vi "Message Handling Loop - UI.vi"(8 "error in":errorcluster, 9 "UI":refnum<queue>, 10 "User Event Bundle":T1) -> (0 "error out":errorcluster)   [LabVIEW 2018]
uses:
  Type Defs/Filter Cluster.ctl
  Support/Message Queue/Message Queue.lvlib
  Support/Message Queue/Enqueue Message (Single).vi
  <vilib>/Utility/error.llb/Error Cluster From Error Code.vi
  <vilib>/ErrorRing/Error Ring.xnode
  Type Defs/UI Loop Data.ctl
  Type Defs/Sorting Methods.ctl
  Type Defs/SR Cluster.ctl
  Type Defs/SR Status.ctl
  Support/User Events/User Events.lvlib
  Support/Message Queue/Message Cluster.ctl
  Type Defs/User Events.ctl
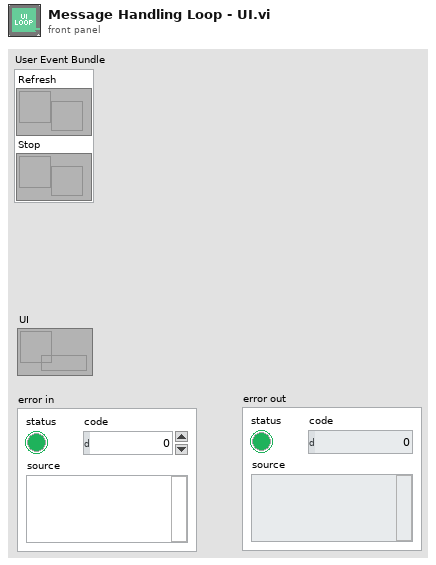
[diagram p1: front panel]
types:
  T1 = typedef "User Events.ctl" = cluster{"Refresh":refnum<user-event>, "Stop":refnum<user-event>}
  T2 = typedef "UI Loop Data.ctl" = cluster{"SR Display List":T3[], "Filter Cluster":T5, "Exit":refnum<vi>, "Main VI":refnum<vi>, "Sorting":T6, "SR Display List":refnum<vi>}
  T3 = typedef "SR Cluster.ctl" = cluster{"Color":u32, "SR Number":i32, "SR Status":T4, "Name":string, "Summary":string, "Last Updated":timestamp, "SR Type":string, "Service Level":string, "Days Open":dbl, "Creation Date":timestamp}
  T4 = typedef "SR Status.ctl" = enum16{"Caller Abandoned", "Created in Error", "Expired", "Forum Resolved AE", "Forum Resolved Customer", "IN WORK", "IN WORK Collab with AES", "IN WORK Collab with PSE", "IN WORK Collab with SE", "IN WORK Customer Added Note", "IN WORK Escalation", "IN WORK Wait on Customer", "Open", "Potentially Resolved", "Presumed Resolved", "RMA Approved for Return", "Resolved", "Passed Off"}
  T5 = typedef "Filter Cluster.ctl" = cluster{"Show Resolved":bool, "Show Potentially Resolved":bool, "Show Passoffs":bool, "Show In Collab":bool}
  T6 = typedef "Sorting Methods.ctl" = enum16{"SR Status", "Most Recent", "SR Type", "SR Number"}
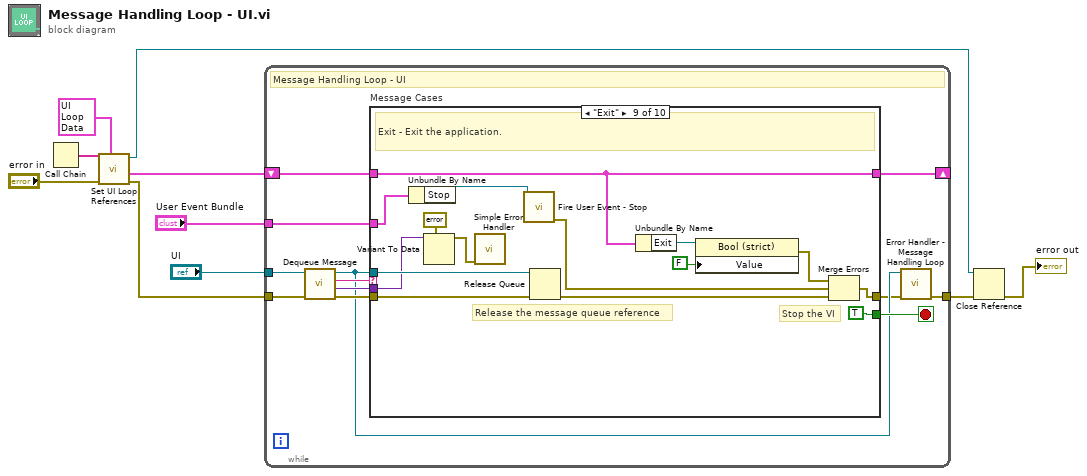
[diagram p0: block diagram]
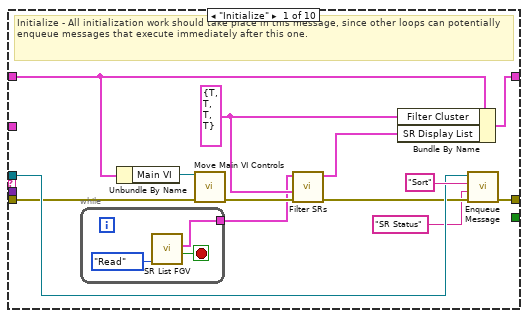
[diagram p2: hidden frame]
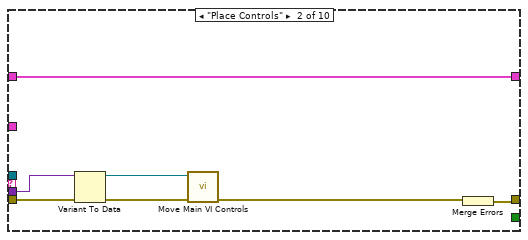
[diagram p3: hidden frame]
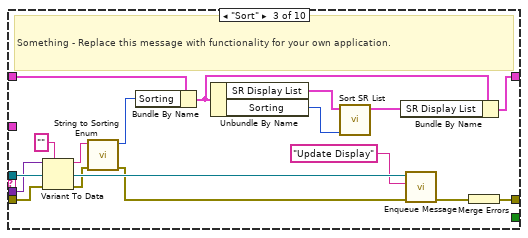
[diagram p4: hidden frame]
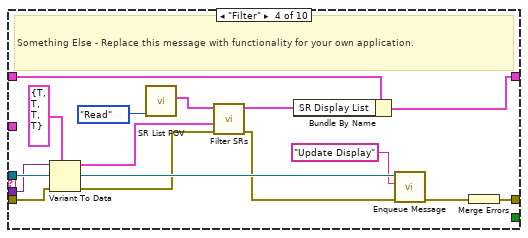
[diagram p5: hidden frame]
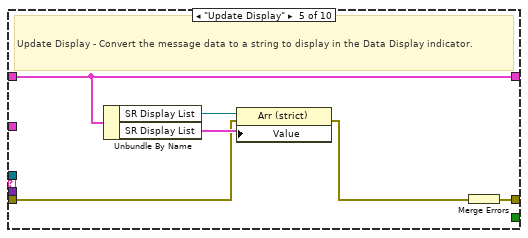
[diagram p6: hidden frame]
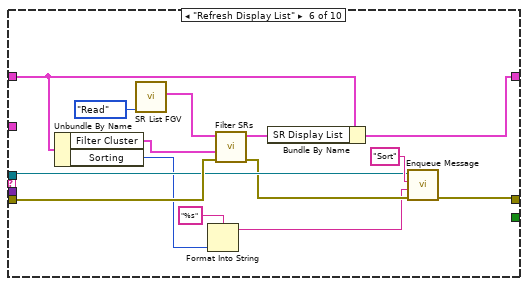
[diagram p7: hidden frame]
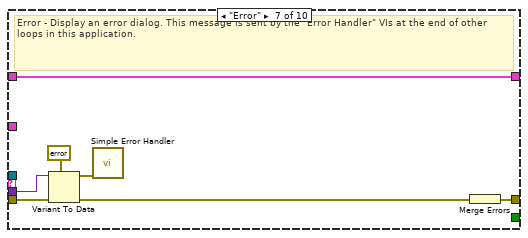
[diagram p8: hidden frame]
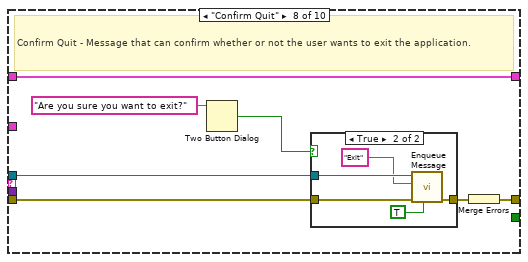
[diagram p9: hidden frame]
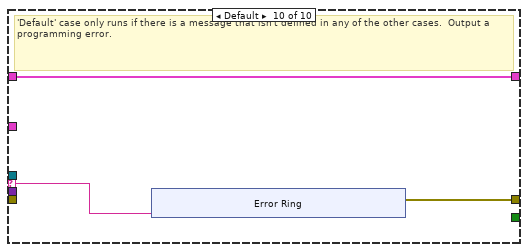
[diagram p11: hidden frame]
diagram:
  n1 = Call Chain() -> (call chain=w4:string[])
  n2 = call "Set UI Loop References.vi"("UI Data in"=T2 {"SR Display List"=[], "Filter Cluster"={"Show Resolved"=TRUE, "Show Potentially Resolved"=TRUE, "Show Passoffs"=TRUE, "Show In Collab"=TRUE}, "Exit"=refnum, "Main VI"=refnum, "Sorting"=enum."SR Status", "SR Display List"=refnum}, "error in (no error)"="error in", "call chain"=w4) -> ("error out"=w8:errorcluster, "UI Data out"=w9:T2, "VI reference out"=w7:refnum<vi>)  [unwired: 6 in]
  n3 = while {
    tunnel: "UI" -> [w15]
    shift-right: [w21] -> _
    shift-left: w9 -> [w22]
    tunnel: w8 -> [w19]
    tunnel: [w13] -> w5
    tunnel: "User Event Bundle" -> [w11]
    stop <- w20 stop-if-true
    # "Message Handling Loop - UI"
    n4 = call "Dequeue Message.vi"("error in (no error)"=w19, "Message Queue"=w15) -> ("error out"=w18:errorcluster, "Message Data"=w16:variant, "Message"=w17:string, "dup Message Queue"=w14:refnum<queue>)  [unwired: 6 in]
    n5 = case "Message Cases" shown="\"Exit\"" w17 {
      selector: w17 -> [_ _ _ _ _ _ _ _ _ w133]
      tunnel: w14 -> [w33 _ w60 w75 _ w91 _ w107 w132 _]
      tunnel: w18 -> [w32 w44 w55 w65 w79 w93 w104 w111 w129 _]
      tunnel: [w35 w40 w62 w77 w83 w89 w98 w109 w122 w134] -> w12
      tunnel: w22 -> [w30 w45 w48 w70 w82 w88 w103 w110 w125 w135]
      tunnel: [w31 w45 w57 w68 w82 w94 w103 w110 w125 w135] -> w21
      tunnel: [_ _ _ _ _ _ _ _ TRUE _] -> w20
      tunnel: w16 -> [_ w42 w56 w66 _ _ w102 _ w126 _]
      tunnel: w11 -> [_ _ _ _ _ _ _ _ w120 _]
      frame "Initialize" {
        w28 = T5 {"Show Resolved"=TRUE, "Show Potentially Resolved"=TRUE, "Show Passoffs"=TRUE, "Show In Collab"=TRUE} ("Filter Cluster")
        # "Initialize - All initialization work should take place in this message, since other loops can potentially enqueue messages that execute immediately after this one."
        n6 = while {
          tunnel: [w37] -> w24
          stop <- w38 stop-if-true
          n7 = call "SR List FGV.vi"("Operation"=enum16{"Initialize", "Write", "Read", "Clear"}."Read") -> ("Updated?"=w38:bool, "list out"=w37:T3[])  [unwired: 9 in]
        }
        n8 = Unbundle By Name(w30) -> ("Main VI"=w29:refnum<vi>)
        n9 = call "Move Main VI Controls.vi"("error in"=w32, "VIRef in"=w29) -> ("error out"=w26:errorcluster)  [unwired: 9 in]
        n10 = call "Filter SRs.vi"("error in"=w26, "Filter Cluster"=w28, "list in"=w24) -> ("error out"=w25:errorcluster, "list out"=w27:T3[])  [unwired: 7 in]
        n11 = Bundle By Name(cluster=w30, "Filter Cluster"=w28, "SR Display List"=w27) -> (w31:T2)
        n12 = call-poly "Enqueue Message.vi"("error in (no error)"=w25, "Message Data"="SR Status" ("Message"), "Message"="Sort", "Message Queue"=w33) -> ("error out"=w35:errorcluster)  [unwired: 6 in, 1 out]
      }
      frame "Place Controls" {
        n13 = Variant To Data(error in=w44, Variant=w42) -> (data=w43:refnum<vi>, error out=w41:errorcluster)  [unwired: 1 in]
        n14 = call "Move Main VI Controls.vi"("error in"=w41, "VIRef in"=w43) -> ("error out"=w39:errorcluster)  [unwired: 9 in]
        n15 = Merge Errors(w39) -> (w40:errorcluster)
      }
      frame "Sort" {
        # "Something - Replace this message with functionality for your own application."
        n16 = Variant To Data(error in=w55, type="", Variant=w56) -> (data=w54:string, error out=w52:errorcluster)
        n17 = call "String to Sorting Enum.vi"("error in"=w52, "string in"=w54) -> ("error out"=w51:errorcluster, "Sorting"=w47:T6)  [unwired: 8 in]
        n18 = Bundle By Name(cluster=w48, "Sorting"=w47) -> (w46:T2)
        n19 = Unbundle By Name(w46) -> ("SR Display List"=w58:T3[], "Sorting"=w49:T6)
        n20 = call "Sort SR List.vi"("Sorting"=w49, "list in"=w58) -> ("list out"=w50:T3[])  [unwired: 9 in]
        n21 = Bundle By Name(cluster=w46, "SR Display List"=w50) -> (w57:T2)
        n22 = call-poly "Enqueue Message.vi"("error in (no error)"=w51, "Message"="Update Display", "Message Queue"=w60) -> ("error out"=w61:errorcluster)  [unwired: 7 in, 1 out]
        n23 = Merge Errors(w61) -> (w62:errorcluster)
      }
      frame "Filter" {
        # "Something Else - Replace this message with functionality for your own application."
        n24 = Variant To Data(error in=w65, type=T5 {"Show Resolved"=TRUE, "Show Potentially Resolved"=TRUE, "Show Passoffs"=TRUE, "Show In Collab"=TRUE} ("Filter Cluster"), Variant=w66) -> (data=w63:T5, error out=w64:errorcluster)
        n25 = call "SR List FGV.vi"("Operation"=enum16{"Initialize", "Write", "Read", "Clear"}."Read") -> ("list out"=w72:T3[])  [unwired: 9 in, 1 out]
        n26 = call "Filter SRs.vi"("error in"=w64, "Filter Cluster"=w63, "list in"=w72) -> ("error out"=w73:errorcluster, "list out"=w69:T3[])  [unwired: 7 in]
        n27 = Bundle By Name(cluster=w70, "SR Display List"=w69) -> (w68:T2)
        n28 = call-poly "Enqueue Message.vi"("error in (no error)"=w73, "Message"="Update Display", "Message Queue"=w75) -> ("error out"=w76:errorcluster)  [unwired: 7 in, 1 out]
        n29 = Merge Errors(w76) -> (w77:errorcluster)
      }
      frame "Update Display" {
        # "Update Display - Convert the message data to a string to display in the Data Display indicator."
        n30 = Unbundle By Name(w82) -> ("SR Display List"=w81:refnum<vi>, "SR Display List"=w80:T3[])
        n31 = property class="Arr (strict)"(reference=w81, error in=w79, "Value"=w80) -> (error out=w78:errorcluster)  [unwired: 1 out]
        n32 = Merge Errors(w78) -> (w83:errorcluster)
      }
      frame "Refresh Display List" {
        n33 = Unbundle By Name(w88) -> ("Filter Cluster"=w85:T5, "Sorting"=w84:T6)
        n34 = call "SR List FGV.vi"("Operation"=enum16{"Initialize", "Write", "Read", "Clear"}."Read") -> ("list out"=w96:T3[])  [unwired: 9 in, 1 out]
        n35 = Format Into String(format string="%s", w84) -> (resulting string=w86:string)  [unwired: 2 in, 1 out]
        n36 = call "Filter SRs.vi"("error in"=w93, "Filter Cluster"=w85, "list in"=w96) -> ("error out"=w90:errorcluster, "list out"=w95:T3[])  [unwired: 7 in]
        n37 = Bundle By Name(cluster=w88, "SR Display List"=w95) -> (w94:T2)
        n38 = call-poly "Enqueue Message.vi"("error in (no error)"=w90, "Message Data"=w86, "Message"="Sort", "Message Queue"=w91) -> ("error out"=w89:errorcluster)  [unwired: 6 in, 1 out]
      }
      frame "Error" {
        # "Error - Display an error dialog. This message is sent by the \"Error Handler\" VIs at the end of other loops in this application."
        n39 = Variant To Data(error in=w104, type=errorcluster {"status"=FALSE, "code"=0, "source"=""} ("error constant"), Variant=w102) -> (data=w100:errorcluster, error out=w99:errorcluster)
        n40 = call <vilib>:"Simple Error Handler.vi"("error in (no error)"=w100) -> ()  [unwired: 4 in, 5 out]
        n41 = Merge Errors(w99) -> (w98:errorcluster)
      }
      frame "Confirm Quit" {
        # "Confirm Quit - Message that can confirm whether or not the user wants to exit the application."
        n42 = Two Button Dialog(message="Are you sure you want to exit?") -> (T button?=w105:bool)  [unwired: 2 in]
        n43 = case shown="True" w105 {
          tunnel: w111 -> [w112 w117]
          tunnel: [w112 w116] -> w108
          tunnel: w107 -> [_ w115]
          frame False {
          }
          frame True {
            n44 = call-poly "Enqueue Message.vi"("Priority Message? (F)"=TRUE, "error in (no error)"=w117, "Message"="Exit", "Message Queue"=w115) -> ("error out"=w116:errorcluster)  [unwired: 6 in, 1 out]
          }
        }
        n45 = Merge Errors(w108) -> (w109:errorcluster)
      }
      frame "Exit" {
        # "Stop the VI"
        # "Release the message queue reference"
        # "Exit - Exit the application."
        n46 = Unbundle By Name(w120) -> ("Stop"=w119:refnum<user-event>)
        n47 = Variant To Data(type=errorcluster {"status"=FALSE, "code"=0, "source"=""} ("error constant"), Variant=w126) -> (data=w127:errorcluster)  [unwired: 1 in, 1 out]
        n48 = call <vilib>:"Simple Error Handler.vi"("error in (no error)"=w127) -> ()  [unwired: 4 in, 5 out]
        n49 = call "Fire User Event - Stop.vi"(11:w119) -> ("error out"=w118:errorcluster)  [unwired: 10 in]
        n50 = Release Queue(queue=w132, error in (no error)=w129) -> (error out=w130:errorcluster)  [unwired: 1 in, 2 out]
        n51 = Unbundle By Name(w125) -> ("Exit"=w121:refnum<vi>)
        n52 = property class="Bool (strict)"(reference=w121, "Value"=FALSE) -> (error out=w123:errorcluster)  [unwired: 1 in, 1 out]
        n53 = Merge Errors(w123, w118, w130) -> (w122:errorcluster)
      }
      frame Default {
        # "'Default' case only runs if there is a message that isn't defined in any of the other cases.  Output a programming error."
        n54 = xnode "Error Ring"("parameter 0"=w133) -> ("error out"=w134:errorcluster)
      }
    }
    n55 = call "Error Handler - Message Handling Loop.vi"("error in (no error)"=w12, "Message Queue"=w14) -> ("dup error in"=w13:errorcluster)  [unwired: 8 in, 1 out]
  }
  n56 = Close Reference(reference=w7, error in (no error)=w5) -> (error out=→"error out":errorcluster)
